vi "Set Cells (2D Row String).vi"(6 "Column (0)":i32, 7 "Values":string[][](array[string]), 8 "error in (no error)":errorcluster, 9 "Row (0)":i32, 10 "Sheet Reference":refnum<k24>) -> (0 "error out":errorcluster, 2 "Sheet Reference out":refnum<k24>)   [LabVIEW 2014]
uses:
  C:/Users/LENOVO/Desktop/CodeSpace GUI/LVExcel/Resources/NPOI 2.1.1 dotnet2/NPOI.dll
  Resources/NPOI 2.1.1 dotnet2/NPOI.dll
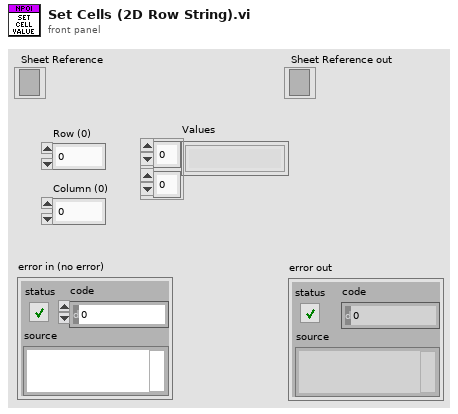
[diagram p1: front panel]
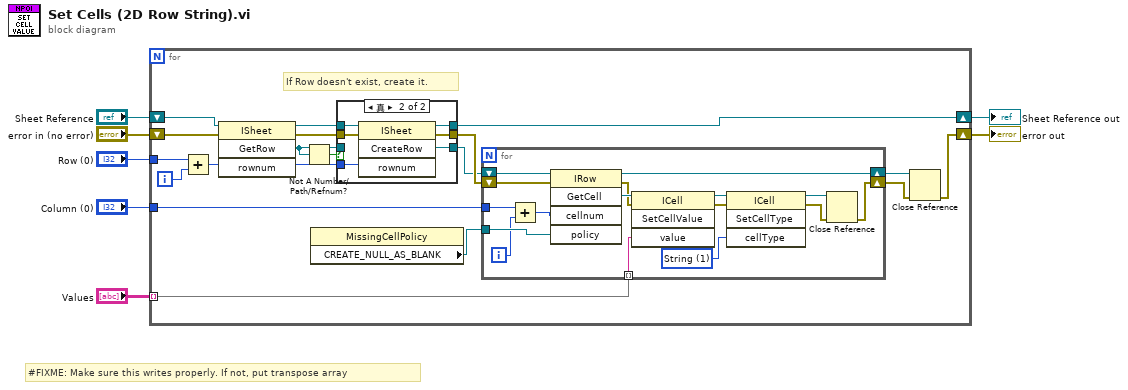
[diagram p0: block diagram]
diagram:
  # "#FIXME: Make sure this writes properly. If not, put transpose array"
  n1 = for {
    tunnel: "Column (0)" -> [w24]
    tunnel: "Row (0)" -> [w15]
    shift-right: [w14] -> w2
    shift-left: "Sheet Reference" -> [w16]
    shift-right: [w22] -> w6
    shift-left: "error in (no error)" -> [w17]
    tunnel: "Values" -> [w10] mode=indexing
    i -> [w8]
    # "If Row doesn't exist, create it."
    n2 = Add(x=w15, y=w8) -> (x+y=w9:i32)
    n3 = invoke class="ISheet" method="GetRow"(reference=w16, error in=w17, "rownum"=w9) -> (reference out=w18:refnum<k24>, error out=w19:errorcluster, "GetRow"=w21:refnum<k24>)  [unwired: 1 in, 1 out]
    n4 = Not A Number/Path/Refnum?(number/path/refnum=w21) -> (NaN/Path/Refnum?=w20:bool)
    n5 = property class="MissingCellPolicy"() -> ("CREATE_NULL_AS_BLANK"=w11:refnum<k24>)  [unwired: 2 in, 2 out]
    n6 = case shown="真" w20 {
      tunnel: w18 -> [w44 w50]
      tunnel: w19 -> [w43 w49]
      tunnel: [w43 w48] -> w13
      tunnel: [w44 w47] -> w14
      tunnel: w9 -> [_ w46]
      tunnel: [w42 w45] -> w12
      tunnel: w21 -> [w42 _]
      frame False {
      }
      frame True {
        n7 = invoke class="ISheet" method="CreateRow"(reference=w50, error in=w49, "rownum"=w46) -> (reference out=w47:refnum<k24>, error out=w48:errorcluster, "CreateRow"=w45:refnum<k24>)  [unwired: 1 in, 1 out]
      }
    }
    n8 = for {
      tunnel: w24 -> [w40]
      tunnel: w11 -> [w34]
      shift-right: [w41] -> w25
      shift-left: w12 -> [w35]
      shift-right: [w37] -> w23
      shift-left: w13 -> [w36]
      tunnel: w10 -> [w26] mode=indexing
      i -> [w32]
      w27 = 1 items=["Numeric"=0, "String"=1, "Formula"=2, "Blank"=3, "Boolean"=4, "Error"=5, "Unknown"=-1] ("cellType")
      n9 = Add(x=w40, y=w32) -> (x+y=w33:i32)
      n10 = invoke class="IRow" method="GetCell"(reference=w35, error in=w36, "cellnum"=w33, "policy"=w34) -> (reference out=w41:refnum<k24>, error out=w38:errorcluster, "GetCell"=w39:refnum<k24>)  [unwired: 1 in, 2 out]
      n11 = invoke class="ICell" method="SetCellValue"(reference=w39, error in=w38, "value"=w26) -> (reference out=w31:refnum<k24>, error out=w30:errorcluster)  [unwired: 1 in, 2 out]
      n12 = invoke class="ICell" method="SetCellType"(reference=w31, error in=w30, "cellType"=w27) -> (reference out=w29:refnum<k24>, error out=w28:errorcluster)  [unwired: 1 in, 2 out]
      n13 = Close Reference(reference=w29, error in (no error)=w28) -> (error out=w37:errorcluster)
    }
    n14 = Close Reference(reference=w25, error in (no error)=w23) -> (error out=w22:errorcluster)
  }
  "Sheet Reference out" <- w2
  "error out" <- w6
